vi "Triggering_no_edit_deletion.vi"(8 "error in (no error)":errorcluster, 11 "working directory":path=path "") -> (0 "error out":errorcluster)   [LabVIEW 2021]
panel:
  out "standard error":string
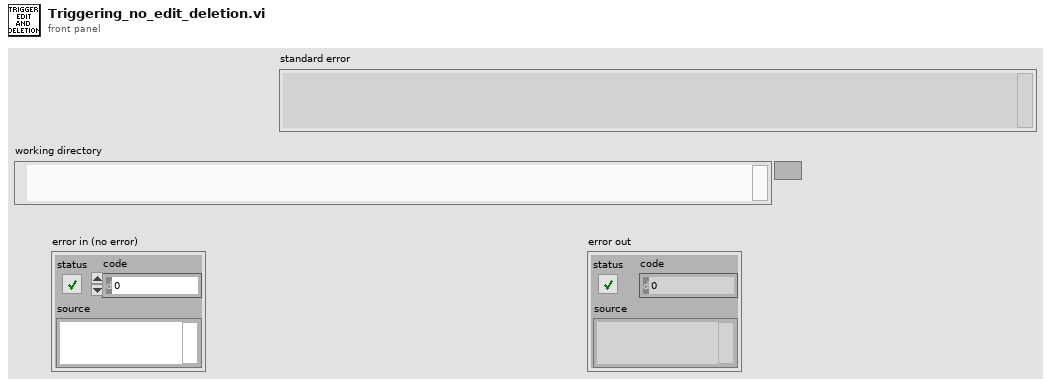
[diagram p1: front panel]
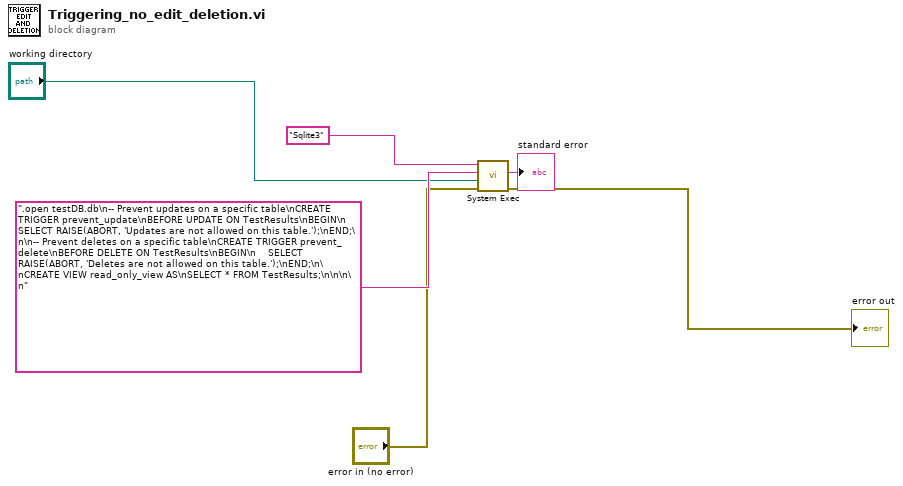
[diagram p0: block diagram]
diagram:
  n1 = call <vilib>:"System Exec.vi"("error in (no error)"="error in (no error)", "working directory"="working directory", "standard input"=".open testDB.db\n-- Prevent updates on a specific table\nCREATE TRIGGER prevent_update\nBEFORE UPDATE ON TestResults\nBEGIN\n    SELECT RAISE(ABORT, 'Updates are not allowed on this table.');\nEND;\n\n-- Prevent deletes on a specific table\nCREATE TRIGGER prevent_delete\nBEFORE DELETE ON TestResults\nBEGIN\n    SELECT RAISE(ABORT, 'Deletes are not allowed on this table.');\nEND;\n\nCREATE VIEW read_only_view AS\nSELECT * FROM TestResults;\n\n\n\n", "command line"="Sqlite3") -> ("error out"=→"error out":errorcluster, "standard error"=→"standard error":string)  [unwired: 4 in, 2 out]
